vi "IsFull.vi"(11 "TypedCircularBuffer in":refnum<class "RotateCircularBuffer.lvclass">) -> (2 "Full?":bool, 3 "TypedCircularBuffer out":refnum<class "RotateCircularBuffer.lvclass">)   [LabVIEW 2024, in "RotateCircularBuffer.lvclass"]
uses:
  RotateCircularBuffer.lvclass
  RotateCircularBuffer.lvclass/RotateCircularBuffer.ctl
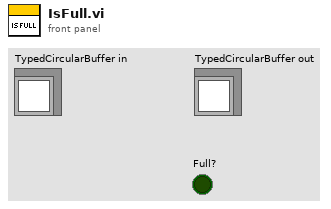
[diagram p1: front panel]
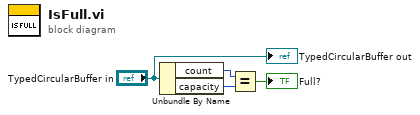
[diagram p0: block diagram]
diagram:
  n1 = Unbundle By Name("TypedCircularBuffer in") -> ("count"=w3:u32, "capacity"=w2:u32)
  n2 = Equal?(x=w3, y=w2) -> (x = y?=→"Full?":bool)
  "TypedCircularBuffer out" <- "TypedCircularBuffer in"
